vi "Wait(sec) text in.vi"(0 "command text in":string[](array[string])) -> (1 "extra wait (sec)":i32 min=0)   [LabVIEW 2020]
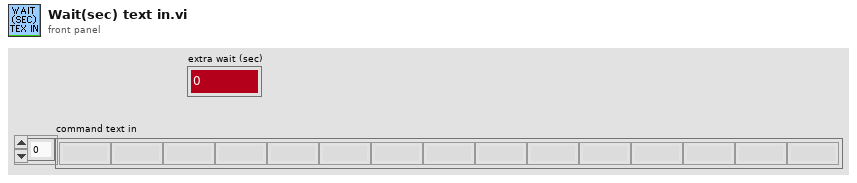
[diagram p1: front panel]
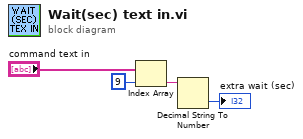
[diagram p0: block diagram]
diagram:
  n1 = Index Array(array="command text in", index=9) -> (element=w1:string)
  n2 = Decimal String To Number(string=w1) -> (number=→"extra wait (sec)":i32)  [unwired: 2 in, 1 out]
